vi "RP hoekcorrelatie-analyse-V2.vi"() -> ()   [LabVIEW 2013]
uses:
  <vilib>/Utility/file.llb/Read From Spreadsheet File (DBL).vi
panel:
  in  "Boolean":bool
  in  "sigma (mrad) 2":dbl
  out "Sum of squared residuals":dbl
  out "output cluster 2":cluster{ext[], ext[]}
  out "XY Graph 5":cluster{ext[], "Array out":ext[]}[](graph)
  out "2d - Acar 4":bool
  out "2d - Acar 3":bool
  out "2d - Acar 2":bool
  in  "1d - Acar":bool caption="2d - Acar or DB"
  out "?":dbl format="%#_3g"
  in  "22Na source radius (mm)":dbl=0.1 min=1e-05 max=3.0
  in  "measurement file\n\n         ??. txt":bool
  out "Fermi energy (eV)":dbl format="%#_3g"
  in  "background \n coincidence counts":dbl min=0.0 max=100.0
  in  "alignment correction":dbl min=-10.0 max=10.0 step=0.0001
  out "XY Graph 4":cluster{ext[], "Array out":ext[]}[](graph)
  in  "stop 4":bool
  in  "collimator afstand\n       (mm)":dbl=500.0 min=100.0 max=1000.0
  in  "spleetbreedte\n      (mm)":dbl=1.0 min=0.1 max=5.0
  out "ZICHT  functie":cluster{"Y":dbl[], "Y":dbl[]}[](graph)
  in  "fraction core\nannihilations":dbl=0.2 min=0.0 max=1.0 step=1e-05
  in  "core width\n   (mrad)":dbl=5.0
  out "core electrons":cluster{"Y":dbl[], "Y":dbl[]}[](graph)
  in  "stop 2":bool
  in  "Fermi angle\n   (mrad)":dbl=7.0
  out "free gas model":cluster{"Y":dbl[], "Y":dbl[]}[](graph)
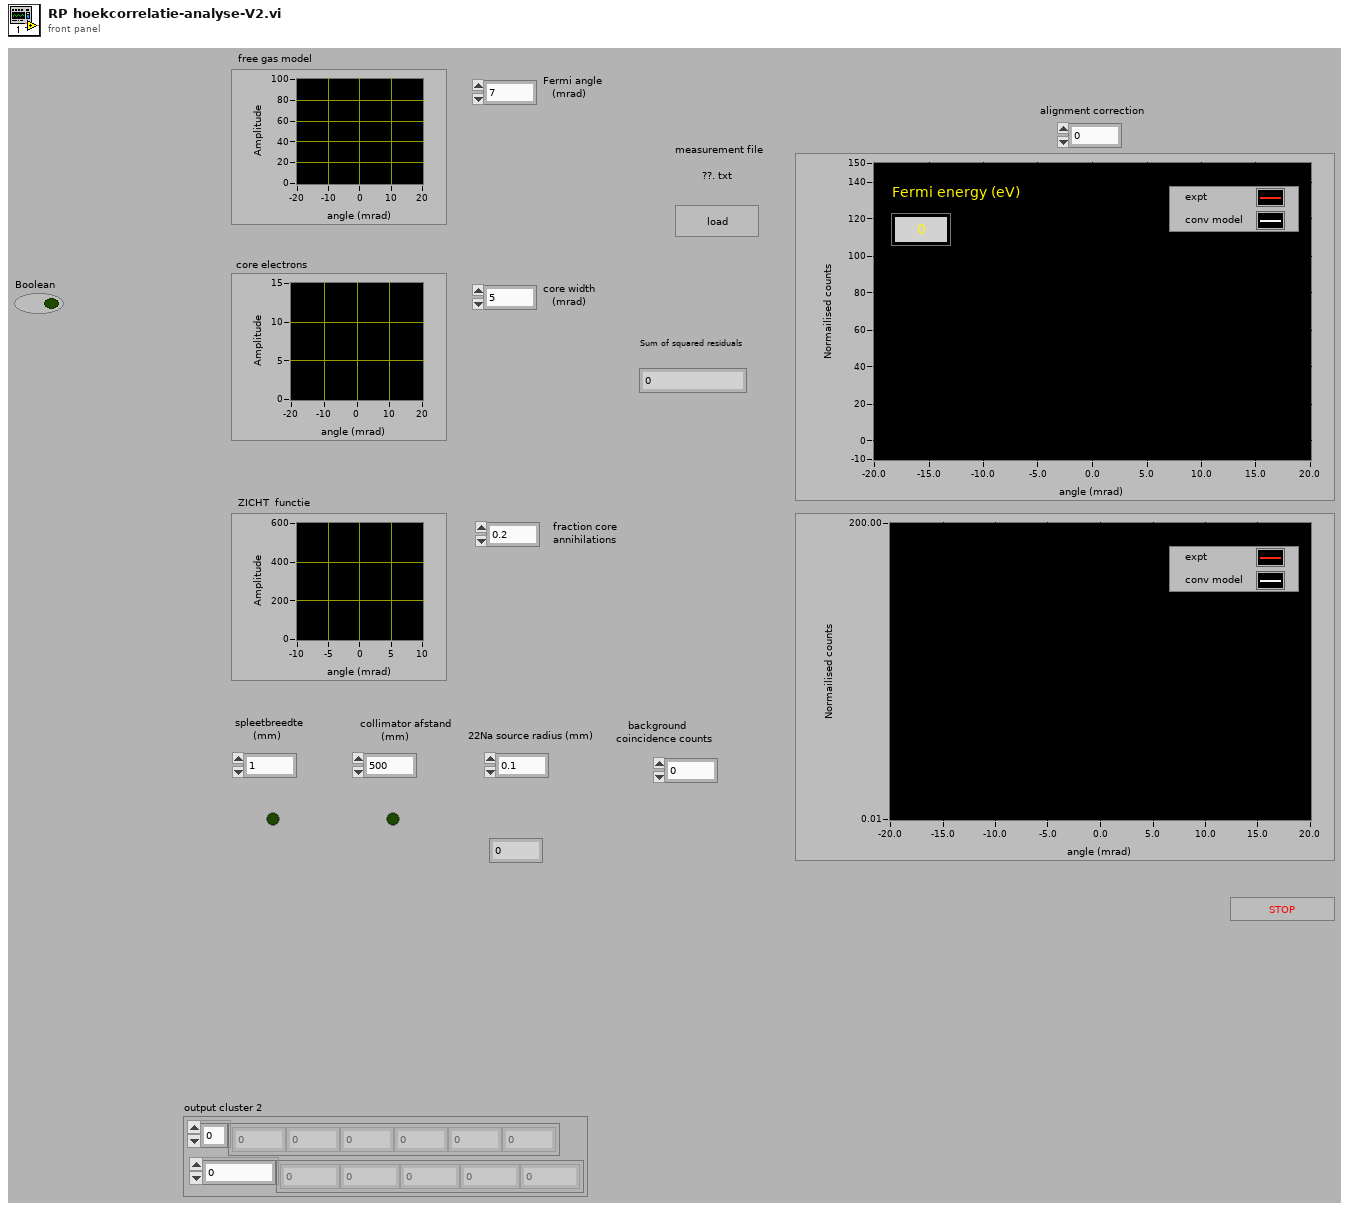
[diagram p1: front panel]
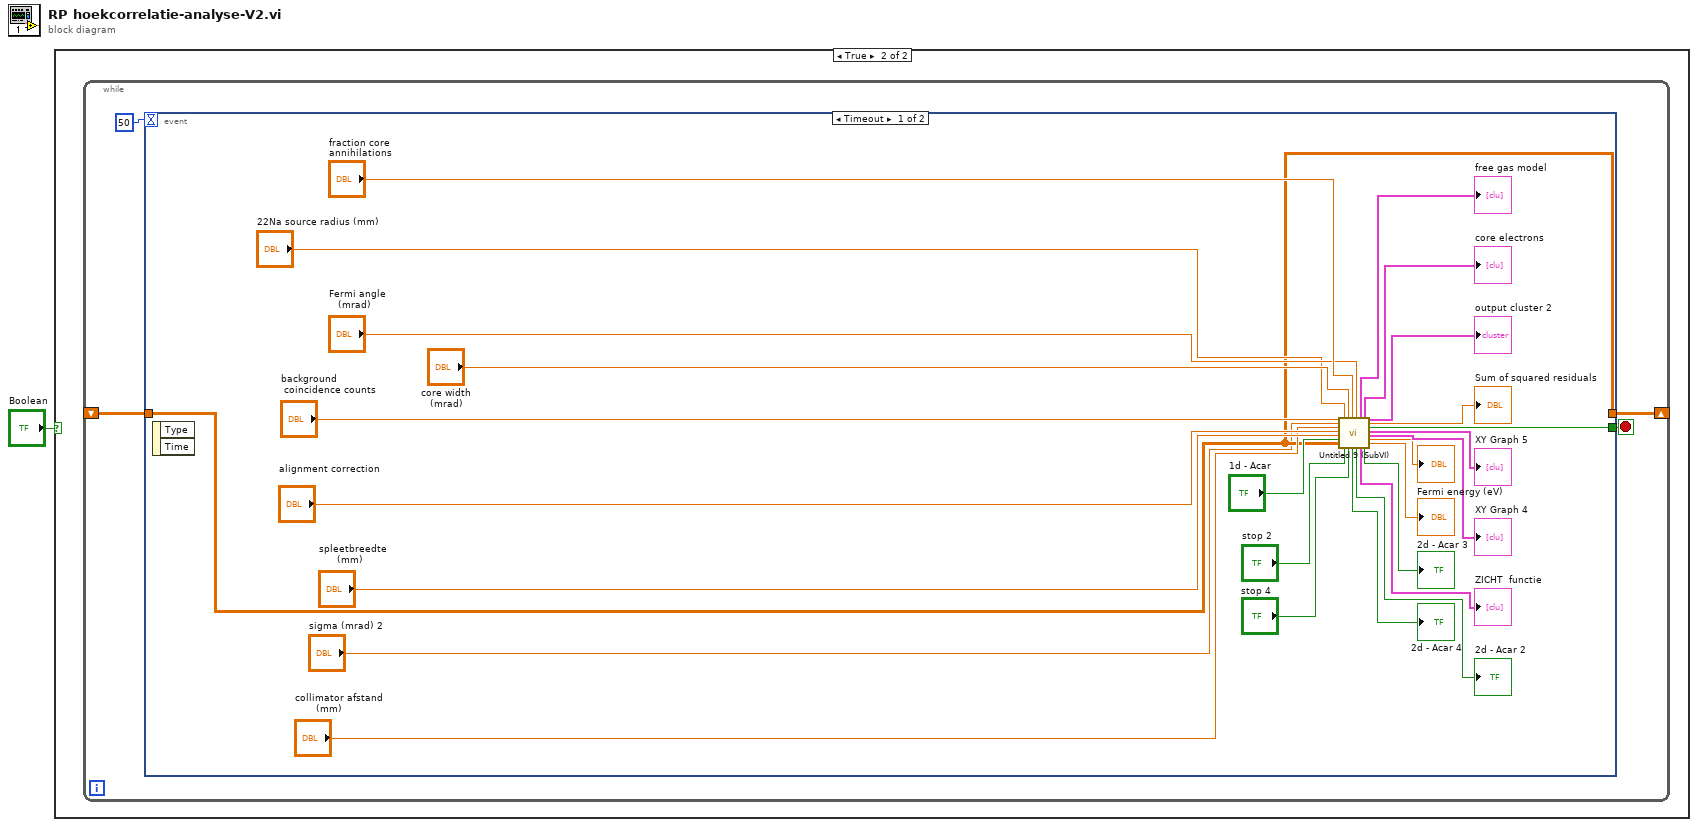
[diagram p0: block diagram]
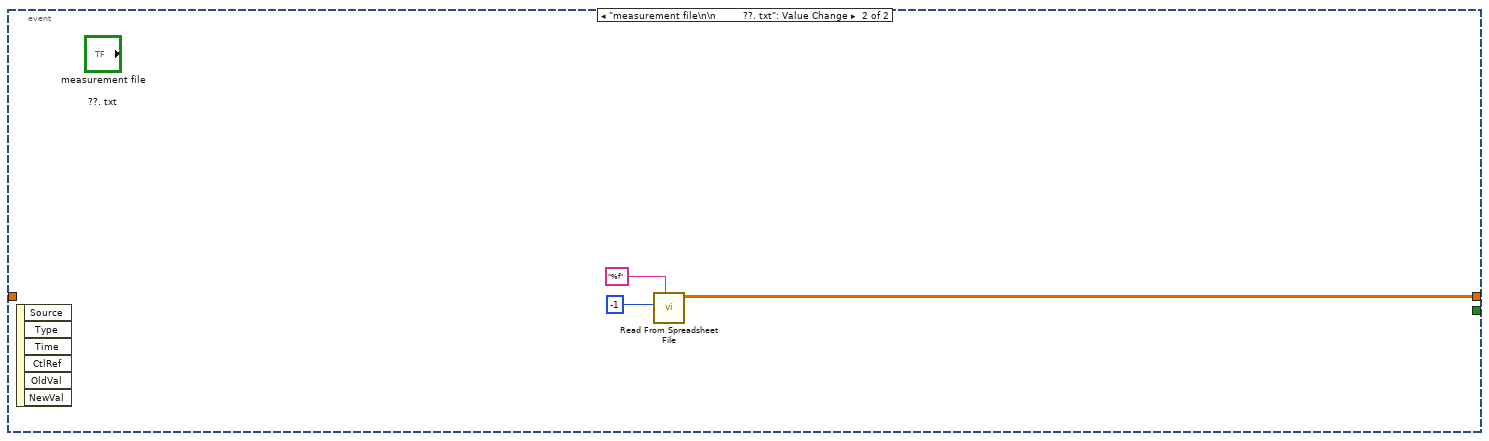
[diagram p3: hidden frame]
diagram:
  n1 = case shown="True" "Boolean" {
    frame False {
    }
    frame True {
      n2 = while {
        shift-right: [w3] -> _
        shift-left: _ -> [w2]
        stop <- w5 stop-if-true
        n3 = event shown="[0] Timeout" {
          selector: _ -> [_ _]
          dyn-events: _ -> [_ _]
          timeout: 50 -> [_ _]
          tunnel: [w31 _] -> w5
          tunnel: [w21 w33] -> w3
          tunnel: w2 -> [w21 _]
          event Timeout {
            n4 = event-data() -> ()  [unwired: 1 in, 2 out]
            n5 = call "Untitled 9 (SubVI).vi"("background \n coincidence counts"="background \n coincidence counts", "sigma (mrad) in"="sigma (mrad) 2", "collimator afstand\n       (mm)"="collimator afstand\n       (mm)", "alignment correction"="alignment correction", "spleetbreedte\n      (mm)"="spleetbreedte\n      (mm)", "1d - Acar"="1d - Acar", "all rows"=w21, "22Na source radius (mm)"="22Na source radius (mm)", "stop in"="stop 2", "core width\n   (mrad)"="core width\n   (mrad)", "stop 4"="stop 4", "fraction core\nannihilations"="fraction core\nannihilations", "Fermi angle\n   (mrad)"="Fermi angle\n   (mrad)") -> ("2d - Acar 4"=→"2d - Acar 4":bool, "2d - Acar 2"=→"2d - Acar 2":bool, "free gas model"=→"free gas model":cluster{"Y":dbl[], "Y":dbl[]}[], "ZICHT  functie"=→"ZICHT  functie":cluster{"Y":dbl[], "Y":dbl[]}[], "core electrons"=→"core electrons":cluster{"Y":dbl[], "Y":dbl[]}[], "2d - Acar 3"=→"2d - Acar 3":bool, "output cluster 2"=→"output cluster 2":cluster{ext[], ext[]}, "Sum of squared residuals"=→"Sum of squared residuals":dbl, "stop 3"=w31:bool, "XY Graph 5"=→"XY Graph 5":cluster{ext[], "Array out":ext[]}[], "XY Graph 4"=→"XY Graph 4":cluster{ext[], "Array out":ext[]}[], 25:→"?":dbl, "Fermi energy (eV)"=→"Fermi energy (eV)":dbl)  [unwired: 2 in]
          }
          event "measurement file\n\n         ??. txt": Value Change {
            n6 = event-data() -> ()  [unwired: 1 in, 6 out]
            n7 = call-poly <vilib>:"Read From Spreadsheet File.vi"("format (%.3f)"="%f", "number of rows (all:-1)"=-1) -> ("all rows"=w33:ext[][])  [unwired: 5 in, 4 out]
          }
        }
      }
    }
  }
